vi "Receive Voltage.vi"(8 "error in (no error)":errorcluster, 10 "Receive Voltage":waveform(dbl)[](array[waveform]), 11 "Get Voltage in":refnum<class "Get Voltage.lvclass">) -> (0 "error out":errorcluster, 3 "Get Voltage out":refnum<class "Get Voltage.lvclass">)   [LabVIEW 2021, in "Get Voltage.lvclass"]
uses:
  Get Voltage.lvclass
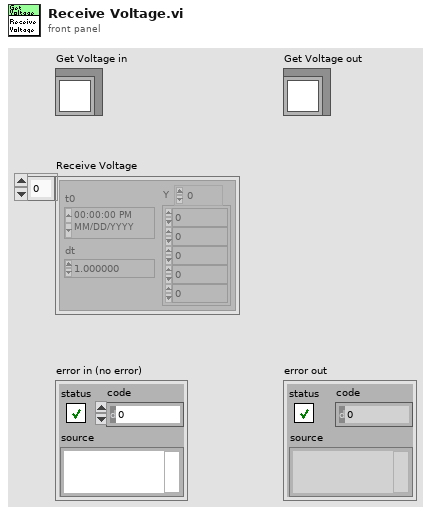
[diagram p1: front panel]
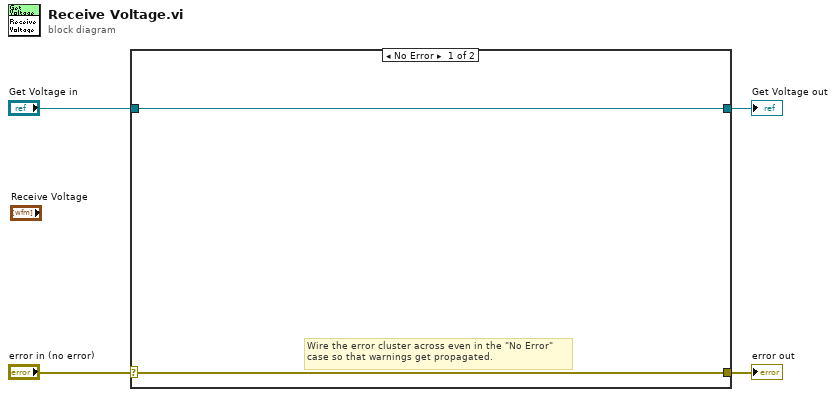
[diagram p0: block diagram]
diagram:
  n1 = case shown="No Error" "error in (no error)" {
    selector: "error in (no error)" -> [w5 w8]
    tunnel: [w5 w8] -> w3
    tunnel: [w6 w7] -> w1
    tunnel: "Get Voltage in" -> [w6 w7]
    frame No Error {
      # "Wire the error cluster across even in the \"No Error\"\ncase so that warnings get propagated."
    }
    frame Error {
    }
  }
  "error out" <- w3
  "Get Voltage out" <- w1
